vi "WhitelistProperties.vi"(9 "white list property names":string[](array[string]), 10 "property names in":string[](array[string]), 11 "property values in":variant[](array[variant])) -> (2 "property names out":string[](array[string]), 3 "property values out":variant[](array[variant]))   [LabVIEW 2017, in "DataExplorerSupport.lvlib"]
uses:
  <vilib>/addons/InsightCM/Utilities/DataExplorerSupport/DataExplorerSupport.lvlib
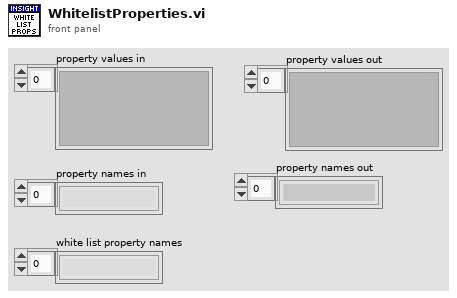
[diagram p1: front panel]
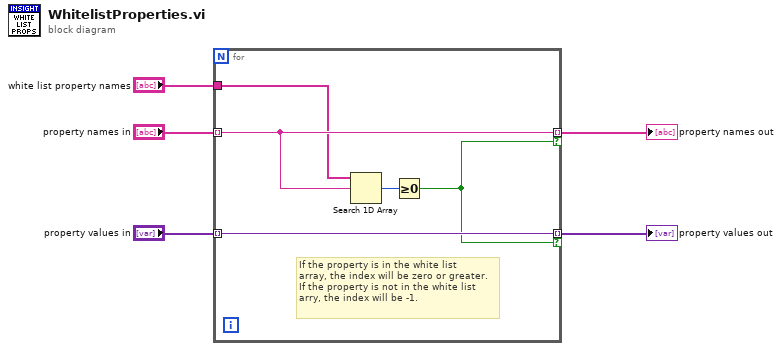
[diagram p0: block diagram]
diagram:
  n1 = for {
    tunnel: "property names in" -> [w9] mode=indexing
    tunnel: "property values in" -> [w8] mode=indexing
    tunnel: [w9] -> w4 mode=indexing if=w7
    tunnel: [w8] -> w2 mode=indexing if=w7
    tunnel: "white list property names" -> [w6]
    # "If the property is in the white list\narray, the index will be zero or greater.\nIf the property is not in the white list\narry, the index will be -1."
    n2 = Search 1D Array(1D array=w6, element=w9) -> (index of element=w10:i32)  [unwired: 1 in]
    n3 = Greater Or Equal To 0?(x=w10) -> (x >= 0?=w7:bool)
  }
  "property values out" <- w2
  "property names out" <- w4
